vi "Initialise Listbox.vi"(8 "error in (no error)":errorcluster, 11 "MCListbox with Checkboxes in":refnum<class "MCListbox with Checkboxes.lvclass">) -> (0 "error out":errorcluster, 3 "MCListbox with Checkboxes out":refnum<class "MCListbox with Checkboxes.lvclass">)   [LabVIEW 2016, in "MCListbox with Checkboxes.lvclass"]
uses:
  MCListbox with Checkboxes.lvclass
  MCListbox with Checkboxes.lvclass/MCListbox with Checkboxes.ctl
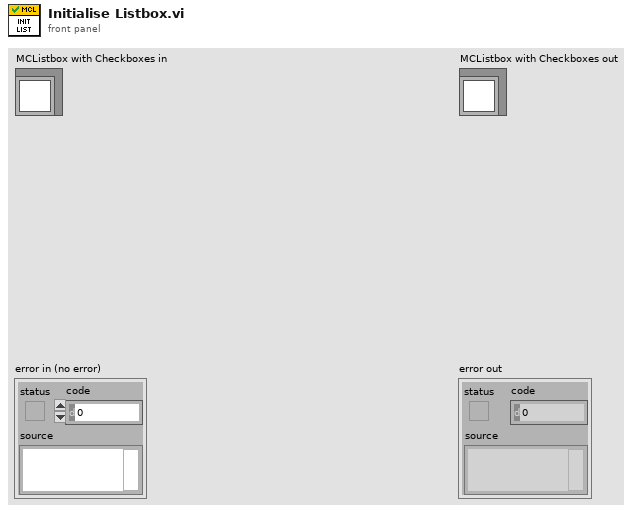
[diagram p1: front panel]
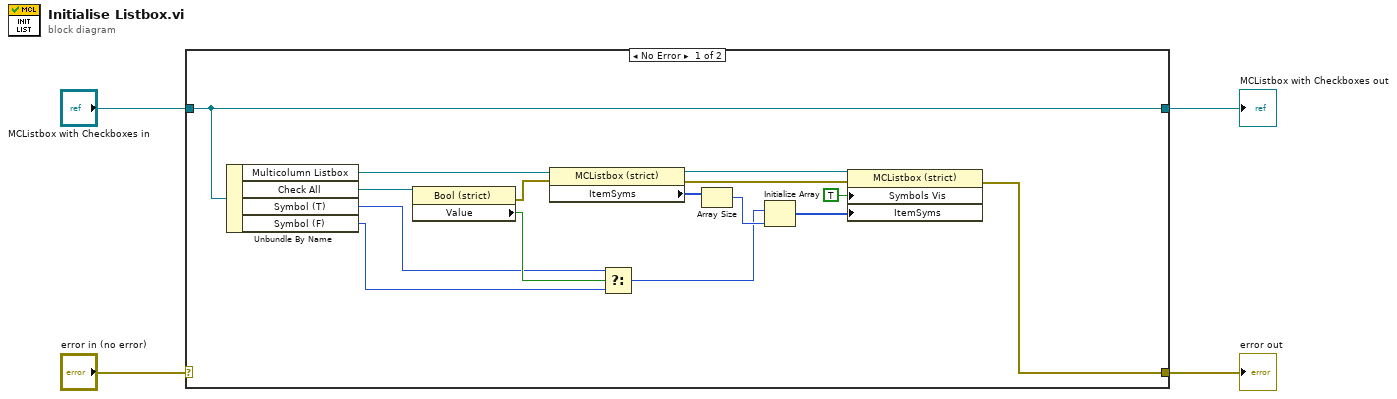
[diagram p0: block diagram]
diagram:
  n1 = case shown="No Error" "error in (no error)" {
    selector: "error in (no error)" -> [_ w21]
    tunnel: [w17 w21] -> w3
    tunnel: [w19 w20] -> w1
    tunnel: "MCListbox with Checkboxes in" -> [w19 w20]
    frame No Error {
      n2 = Unbundle By Name(w19) -> ("Multicolumn Listbox"=w12:refnum<vi>, "Check All"=w16:refnum<vi>, "Symbol (T)"=w14:i32, "Symbol (F)"=w13:i32)
      n3 = property class="Bool (strict)"(reference=w16) -> (error out=w11:errorcluster, "Value"=w15:bool)  [unwired: 1 in, 1 out]
      n4 = property class="MCListbox (strict)"(reference=w12, error in=w11) -> (reference out=w6:refnum<vi>, error out=w5:errorcluster, "ItemSyms"=w10:i32[])
      n5 = Select(t=w14, s=w15, f=w13) -> (s? t:f=w8:i32)
      n6 = Array Size(array=w10) -> (size(s)=w9:i32)
      n7 = Initialize Array(w8, w9) -> (w7:i32[])
      n8 = property class="MCListbox (strict)"(reference=w6, error in=w5, "Symbols Vis"=TRUE ("Visible Items:Symbols Visible"), "ItemSyms"=w7) -> (error out=w17:errorcluster)  [unwired: 1 out]
    }
    frame Error {
    }
  }
  "error out" <- w3
  "MCListbox with Checkboxes out" <- w1
